vi "Disabled - Constant System (SubVI).vi"(10 "Load Constants":bool) -> (2 "error out":errorcluster, 3 "Constant Cluster out":T1 {"32. shooterHoodAngleRange" format="%_6f"; "31. turretAngleRange" format="%_6f"; "30. shooterVelocityLowerLimit" format="%_6f"; "29. shooterVelocityUpperLimit" format="%_6f"; "28. Robot Track Width (inches)" format="%_6f"; "27. Shooter Spin Up Speed (RPM)" format="%_6f"; "26. Climb Down Speed %" format="%_6f"; "25. Climb Up Speed %" format="%_6f"; "24. wallShooterVelocity" format="%_6f"; "23. Intake Spit Speed %" format="%_6f"; "22. Intake Suck Speed %" format="%_6f"; "21. CP Wheel Diameter" format="%_6f"; "20. Clockwise CP Fudge" format="%_6f"; "19. CouterClockwise CP Fudge" format="%_6f"; "18. Inches per Sector" format="%_6f"; "17. Ticks/Rotation Neo 550" format="%_6f"; "16. Control Panel Wheel Diameter" format="%_6f"; "15. Center-Center Sector Distance" format="%_6f"; "14. Inches / Tick Drivetrain" format="%_6f"; "13. Auton I Output Limit Drive Straight Gain" format="%_6f"; "12. Auton Deriv Drive Straight Gain" format="%_6f"; "11. Auton Int Drive Straight Gain" format="%_6f"; "10. Auton Prop Drive Straight Gain" format="%_6f"; "9. Auton I Output Limit Turn Gain" format="%_6f"; "8. Auton Deriv Turn Gain" format="%_6f"; "7. Auton Int Turn Gain" format="%_6f"; "1. Auton Prop Drive Gain" format="%_6f"; "2. Auton Int Drive Gain" format="%_6f"; "3. Auton Deriv Drive Gain" format="%_6f"; "4. I Output Drive  Limit" format="%_6f"; "5. Auto Drive Cheat (%)" format="%_6f"; "6. Auton Prop Turn Gain" format="%_6f"})   [LabVIEW 2019]
uses:
  Disabled - Constant Cluster Typedef.ctl
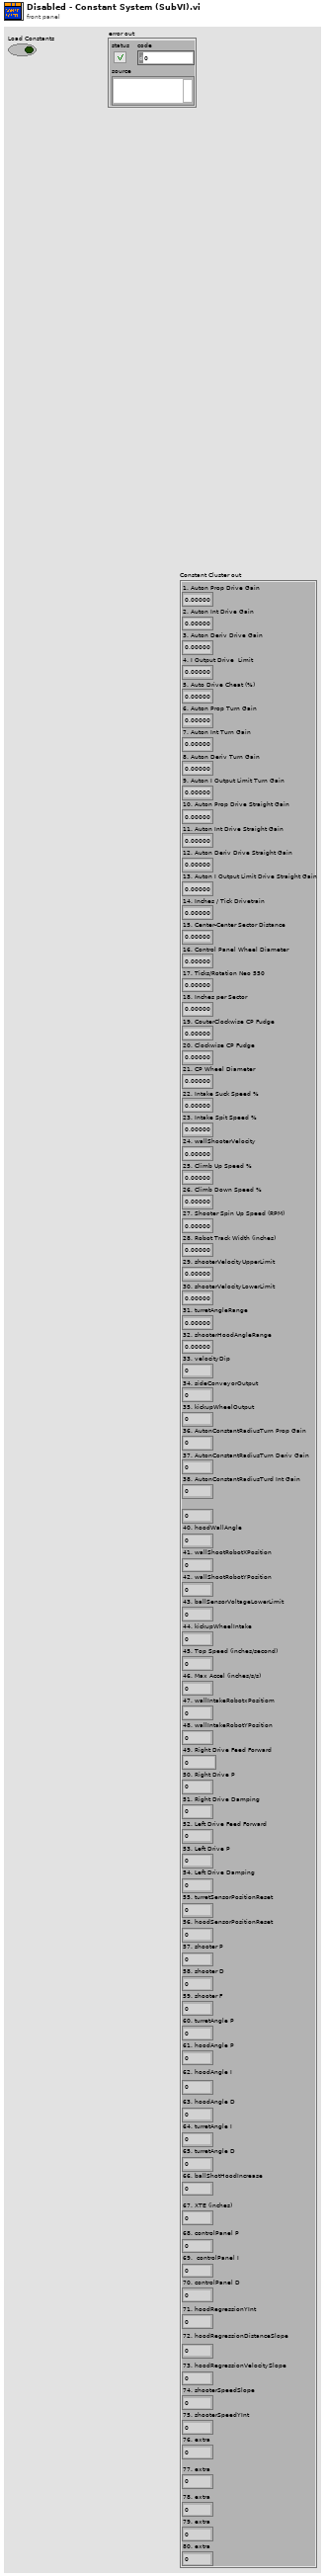
[diagram p1: front panel]
types:
  T1 = typedef "Disabled - Constant Cluster Typedef.ctl" = cluster{"1. Auton Prop Drive Gain":dbl, "2. Auton Int Drive Gain":dbl, "3. Auton Deriv Drive Gain":dbl, "4. I Output Drive  Limit":dbl, "5. Auto Drive Cheat (%)":dbl, "6. Auton Prop Turn Gain":dbl, "7. Auton Int Turn Gain":dbl, "8. Auton Deriv Turn Gain":dbl, "9. Auton I Output Limit Turn Gain":dbl, "10. Auton Prop Drive Straight Gain":dbl, "11. Auton Int Drive Straight Gain":dbl, "12. Auton Deriv Drive Straight Gain":dbl, "13. Auton I Output Limit Drive Straight Gain":dbl, "14. Inches / Tick Drivetrain":dbl, "15. Center-Center Sector Distance":dbl, "16. Control Panel Wheel Diameter":dbl, "17. Ticks/Rotation Neo 550":dbl, "18. Inches per Sector":dbl, "19. CouterClockwise CP Fudge":dbl, "20. Clockwise CP Fudge":dbl, "21. CP Wheel Diameter":dbl, "22. Intake Suck Speed %":dbl, "23. Intake Spit Speed %":dbl, "24. wallShooterVelocity":dbl, "25. Climb Up Speed %":dbl, "26. Climb Down Speed %":dbl, "27. Shooter Spin Up Speed (RPM)":dbl, "28. Robot Track Width (inches)":dbl, "29. shooterVelocityUpperLimit":dbl, "30. shooterVelocityLowerLimit":dbl, "31. turretAngleRange":dbl, "32. shooterHoodAngleRange":dbl, "33. velocityDip":dbl, "34. sideConveyorOutput":dbl, "35. kickupWheelOutput":dbl, "36. AutonConstantRadiusTurn Prop Gain":dbl, "37. AutonConstantRadiusTurn Deriv Gain":dbl, "38. AutonConstantRadiusTurd Int Gain":dbl, "39. turretWallAngle":dbl, "40. hoodWallAngle":dbl, "41. wallShootRobotXPosition":dbl, "42. wallShootRobotYPosition":dbl, "43. ballSensorVoltageLowerLimit":dbl, "44. kickupWheelIntake":dbl, "45. Top Speed (inches/second)":dbl, "46. Max Accel (inches/s/s)":dbl, "47. wallIntakeRobotxPositiom":dbl, "48. wallIntakeRobotYPosition":dbl, "49. Right Drive Feed Forward":dbl, "50. Right Drive P":dbl, "51. Right Drive Damping":dbl, "52. Left Drive Feed Forward":dbl, "53. Left Drive P":dbl, "54. Left Drive Damping":dbl, "55. turretSensorPositionReset":dbl, "56. hoodSensorPositionReset":dbl, "57. shooter P":dbl, "58. shooter D":dbl, "59. shooter F":dbl, "60. turretAngle P":dbl, "61. hoodAngle P":dbl, "62. hoodAngle I":dbl, "63. hoodAngle D":dbl, "64. turretAngle I":dbl, "65. turretAngle D":dbl, "66. ballShotHoodIncrease":dbl, "67. XTE (inches)":dbl, "68. controlPanel P":dbl, "69.  controlPanel I":dbl, "70. controlPanel D":dbl, "71. hoodRegressionYInt":dbl, "72. hoodRegressionDistanceSlope":dbl, "73. hoodRegressionVelocitySlope":dbl, "74. shooterSpeedSlope":dbl, "75. shooterSpeedYInt":dbl, "76. extra":dbl, "77. extra":dbl, "78. extra":dbl, "79. extra":dbl, "80. extra":dbl}
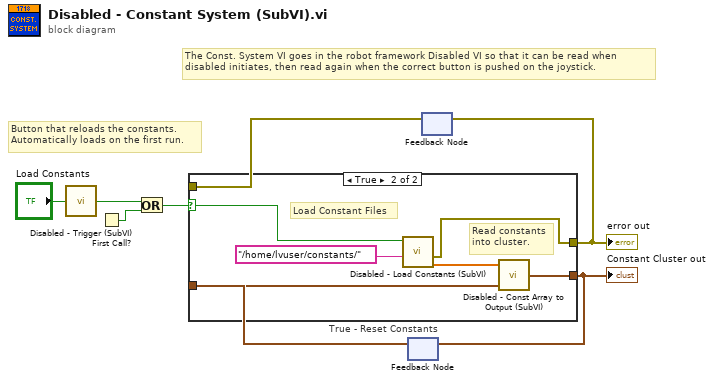
[diagram p0: block diagram]
diagram:
  # "The Const. System VI goes in the robot framework Disabled VI so that it can be read when\ndisabled initiates, then read again when the correct button is pushed on the joystick."
  # "Button that reloads the constants.\nAutomatically loads on the first run."
  n1 = call "Disabled - Trigger (SubVI).vi"("Trigger"="Load Constants") -> ("Trigger Output"=w3:bool)
  n2 = First Call?() -> (First Call?: T/F=w5:bool)
  n3 = Or(x=w3, y=w5) -> (x .or. y?=w4:bool)
  n4 = feedback #1() -> (w6:T1)  [unwired: 1 in]
  n5 = feedback #2() -> (w1:errorcluster)  [unwired: 1 in]
  n6 = case "True - Reset Constants" shown="True" w4 {
    selector: w4 -> [_ w13]
    tunnel: [w10 w15] -> w7
    tunnel: w6 -> [w10 w12]
    tunnel: [w9 w11] -> w2
    tunnel: w1 -> [w9 _]
    frame False {
    }
    frame True {
      # "Read constants\ninto cluster."
      # "Load Constant Files"
      n7 = call "Disabled - Load Constants (SubVI).vi"("Robot Path"="/home/lvuser/constants/", "Force Reload"=w13) -> ("Constants Numeric\nArray"=w16:dbl[], "error out"=w11:errorcluster)  [unwired: 7 in, 1 out]
      n8 = call "Disabled - Const Array to Output (SubVI).vi"("Constant cluster"=w12, "Constants Numeric Array"=w16) -> ("Constant cluster output"=w15:T1)  [unwired: 2 in]
    }
  }
  "Constant Cluster out" <- w7
  "error out" <- w2
  n9 = feedback-in #1(w7) -> ()
  n10 = feedback-in #2(w2) -> ()
